vi "Get Ctrl Refnum.vi"(8 "error in (no error)":errorcluster, 11 "Ctrl Refnum Column in":refnum<class "Ctrl Refnum Column.lvclass">) -> (0 "error out":errorcluster, 2 "Ctl Refnum":refnum<vi>, 3 "Ctrl Refnum Column out":refnum<class "Ctrl Refnum Column.lvclass">)   [LabVIEW 2020, in "Basic Fields.lvlib" / "Ctrl Refnum Column.lvclass"]
uses:
  Ctrl Refnum Column.lvclass
  Ctrl Refnum Column.lvclass/Ctrl Refnum Column.ctl
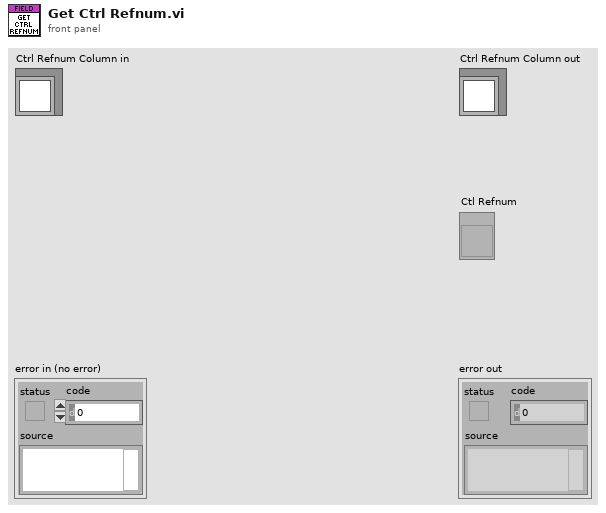
[diagram p1: front panel]
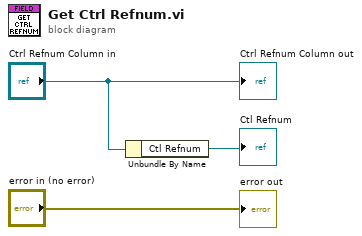
[diagram p0: block diagram]
diagram:
  n1 = Unbundle By Name("Ctrl Refnum Column in") -> ("Ctl Refnum"=→"Ctl Refnum":refnum<vi>)
  "error out" <- "error in (no error)"
  "Ctrl Refnum Column out" <- "Ctrl Refnum Column in"
